vi "SysDef.Create.vi"(8 "error in (no error)":errorcluster, 10 "Configuration":T1={"Name"="", "Description"="", "Diagnostics Basic Configuraiton"={"CAN Interface"=enum."CAN0", "Baud Rate"=0, "Diagnostic Protocol"=enum."GMLAN", "Transport Protocol"=enum."ISO TP - Normal Mode", "Transmit ID"=0, "Receive ID"=0, "Transmit Extension"=0, "Receive Extension"=0, "Receive UUDT ID"=0, "Enable Stream"=TRUE, "VW TP Channel ID"=0, "Security"={"Source DLL Path"=path "", "Security Level"=1, "Target DLL Path"=path ""}, "Fill Frame"=FALSE, "Fill Byte"=255, "Termination"=FALSE}, "DID Outputs"={"Description"="", "Frames"=[]}, "DID Inputs"={"Description"="", "Frames"=[]}, "PID Outputs"={"Description"="", "Frames"=[]}, "PID Inputs"={"Description"="", "Frames"=[]}, "DPIDs"={"Description"="", "DPIDs"=[]}, "DTC"={"Description"="", "DTC descriptor"={"DTC Byte Length"=2, "Status Byte Length"=1, "Add Data Byte Length"=1, "Byte Order"=enum."Motorola"}, "DTC Control"={"Description"="", "Signals"=[]}, "Created DTCs"=0}, "NI 986x Support"={"Enable"=FALSE, "RIO Device"=0, "Bitfile"=path ""}, "Commands"={"Description"=""}, "Status"={"Description"=""}, "IO Controls"={"Description"="", "IO Control Array"=[]}, "Routines"={"Description"="", "Routine Array"=[]}, "Memory Outputs"={"Description"="", "Frames"=[]}, "Memory Inputs"={"Description"="", "Frames"=[]}, "User Defined"={"Description"="", "Groups"=[]}} {"DID Outputs"."Frames"."Signals"."Byte Order" items=["Little Endian", "Big Endian"]; "DID Outputs"."Frames"."Signals"."Data Type" items=["Signed", "Unsigned", "IEEE Float"]; "Memory Inputs"."Frames"."Signals"."Byte Order" items=["Little Endian", "Big Endian"]; "Memory Inputs"."Frames"."Signals"."Data Type" items=["Signed", "Unsigned", "IEEE Float"]; "Memory Outputs"."Frames"."Signals"."Byte Order" items=["Little Endian", "Big Endian"]; "Memory Outputs"."Frames"."Signals"."Data Type" items=["Signed", "Unsigned", "IEEE Float"]; "Routines"."Routine Array"."Stop Parameters"."Response"."Byte Order" items=["Little Endian", "Big Endian"]; "Routines"."Routine Array"."Stop Parameters"."Response"."Data Type" items=["Signed", "Unsigned", "IEEE Float"]; "Routines"."Routine Array"."Stop Parameters"."Cmd"."Byte Order" items=["Little Endian", "Big Endian"]; "Routines"."Routine Array"."Stop Parameters"."Cmd"."Data Type" items=["Signed", "Unsigned", "IEEE Float"]; "Routines"."Routine Array"."Request Parameters"."Response"."Byte Order" items=["Little Endian", "Big Endian"]; "Routines"."Routine Array"."Request Parameters"."Response"."Data Type" items=["Signed", "Unsigned", "IEEE Float"]; "Routines"."Routine Array"."Request Parameters"."Cmd"."Byte Order" items=["Little Endian", "Big Endian"]; "Routines"."Routine Array"."Request Parameters"."Cmd"."Data Type" items=["Signed", "Unsigned", "IEEE Float"]; "Routines"."Routine Array"."Start Parameters"."Response"."Byte Order" items=["Little Endian", "Big Endian"]; "Routines"."Routine Array"."Start Parameters"."Response"."Data Type" items=["Signed", "Unsigned", "IEEE Float"]; "Routines"."Routine Array"."Start Parameters"."Cmd"."Byte Order" items=["Little Endian", "Big Endian"]; "Routines"."Routine Array"."Start Parameters"."Cmd"."Data Type" items=["Signed", "Unsigned", "IEEE Float"]; "IO Controls"."IO Control Array"."Signals"."Response"."Byte Order" items=["Little Endian", "Big Endian"]; "IO Controls"."IO Control Array"."Signals"."Response"."Data Type" items=["Signed", "Unsigned", "IEEE Float"]; "IO Controls"."IO Control Array"."Signals"."Cmd"."Byte Order" items=["Little Endian", "Big Endian"]; "IO Controls"."IO Control Array"."Signals"."Cmd"."Data Type" items=["Signed", "Unsigned", "IEEE Float"]; "DTC"."DTC Control"."Signals"."Byte Order" items=["Little Endian", "Big Endian"]; "DTC"."DTC Control"."Signals"."Data Type" items=["Signed", "Unsigned", "IEEE Float"]; "Diagnostics Basic Configuraiton"."Fill Byte" format="%.0x"; "Diagnostics Basic Configuraiton"."VW TP Channel ID" format="%.0x"; "Diagnostics Basic Configuraiton"."Receive UUDT ID" format="%.0x"; "Diagnostics Basic Configuraiton"."Receive Extension" format="%.0x"; "Diagnostics Basic Configuraiton"."Transmit Extension" format="%.0x"; "Diagnostics Basic Configuraiton"."Receive ID" format="%.0x"; "Diagnostics Basic Configuraiton"."Transmit ID" format="%.0x"; "DID Inputs"."Frames"."Signals"."Byte Order" items=["Little Endian", "Big Endian"]; "DID Inputs"."Frames"."Signals"."Data Type" items=["Signed", "Unsigned", "IEEE Float"]; "PID Inputs"."Frames"."Signals"."Byte Order" items=["Little Endian", "Big Endian"]; "PID Inputs"."Frames"."Signals"."Data Type" items=["Signed", "Unsigned", "IEEE Float"]; "PID Outputs"."Frames"."Signals"."Byte Order" items=["Little Endian", "Big Endian"]; "PID Outputs"."Frames"."Signals"."Data Type" items=["Signed", "Unsigned", "IEEE Float"]}, 11 "Device Item Ref in":T28 format="%.0x") -> (0 "error out":errorcluster, 3 "Device Item Ref out":T28 format="%.0x")   [LabVIEW 2015, in "Diagnostics Addon System Explorer.lvlib"]
uses:
  Diagnostics Addon System Explorer.lvlib
  <vilib>/NI Veristand/Custom Device API/Custom Device Item Ref.ctl
  Types/SysDef.Export.ctl
  Shared/Types/CAN.ctl
  Shared/Types/CAN.Interface.ctl
  Shared/Types/Protocol.ctl
  Shared/Types/Transport.ctl
  Shared/Types/Security.ctl
  Types/Frames.Export.ctl
  Types/Frame.Export.ctl
  Shared/Types/Signal.ctl
  Types/DPIDs.Export.ctl
  Types/DPID.Export.ctl
  Shared/Types/DPID.ctl
  Shared/Types/DPID.Rate.ctl
  Types/DTC.Export.ctl
  Shared/Types/DTCDescriptor.ctl
  Types/DTCControl.Export.ctl
  Shared/Types/986x.ctl
  Types/Command.Export.ctl
  Types/Status.Export.ctl
  Types/IOControls.Export.ctl
  Types/IO.Export.ctl
  Types/CmdResp.Export.ctl
  Types/Routines.Export.ctl
  Types/Routine.Export.ctl
  Types/UserDefined.Export.ctl
  Types/UserDefined.Group.Export.ctl
  Types/UserDefined.Group.Message.Export.ctl
  Types/FG.Action.ctl
  <vilib>/NI Veristand/Custom Device API/Custom Device Channel.ctl
  <vilib>/NI Veristand/Custom Device API/Custom Device Channel Type.ctl
  Shared/Types/Type.ctl
  FileDependency.Create.vi
  Name.Create.vi
  ID.FG.vi
  ReadSignal.Create.vi
  <vilib>/NI Veristand/Custom Device API/NI VeriStand - Get Item Property.vi
  <vilib>/NI Veristand/Custom Device API/Get Item Property (U32).vi
  <vilib>/NI Veristand/Custom Device API/NI VeriStand - Set Item Property.vi
  <vilib>/NI Veristand/Custom Device API/Set Item Property (U32).vi
  Shared/SubVIs/Constants.vi
  <vilib>/NI Veristand/Custom Device API/Get Item Property (I32).vi
  <vilib>/NI Veristand/Custom Device API/Set Item Property (I32).vi
  <vilib>/NI Veristand/Custom Device API/Set Item Property (Boolean).vi
  <vilib>/NI Veristand/Custom Device API/NI VeriStand - Remove Item Property.vi
  <vilib>/NI Veristand/Custom Device API/Set Item Property (Dependent File).vi
  <vilib>/Utility/MD5Checksum.llb/MD5Checksum File.vi
  <vilib>/NI Veristand/Custom Device API/Get Item Property (Boolean).vi
  FileDependency.Get.Target Path.vi
  <vilib>/NI Veristand/Custom Device API/Custom Device API.lvlib
  Shared/Diagnostics Addon Shared.lvlib
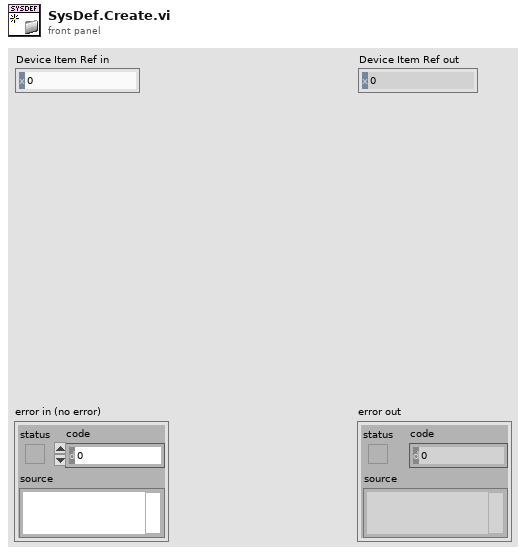
[diagram p1: front panel]
types:
  T1 = typedef "Diagnostics Addon System Explorer.lvlib/SysDef.Export.ctl" = cluster{"Name":string, "Description":string, "Diagnostics Basic Configuraiton":T2, "DID Outputs":T7, "DID Inputs":T7, "PID Outputs":T7, "PID Inputs":T7, "DPIDs":T10, "DTC":T14, "NI 986x Support":T17, "Commands":T18, "Status":T19, "IO Controls":T20, "Routines":T23, "Memory Outputs":T7, "Memory Inputs":T7, "User Defined":T25}
  T2 = typedef "Diagnostics Addon Shared.lvlib/CAN.ctl" = cluster{"CAN Interface":T3, "Baud Rate":u32, "Diagnostic Protocol":T4, "Transport Protocol":T5, "Transmit ID":u32, "Receive ID":u32, "Transmit Extension":u8, "Receive Extension":u8, "Receive UUDT ID":u32, "Enable Stream":bool, "VW TP Channel ID":u32, "Security":T6, "Fill Frame":bool, "Fill Byte":u8, "Termination":bool}
  T3 = typedef "Diagnostics Addon Shared.lvlib/CAN.Interface.ctl" = enum16{"CAN0", "CAN1", "CAN2", "CAN3", "CAN4", "CAN5", "CAN6", "CAN7", "CAN8", "CAN9", "CAN10", "CAN11", "CAN12", "CAN13", "CAN14", "CAN15", "CAN16", "CAN17", "CAN18", "CAN19", "CAN20", "CAN21", "CAN22", "CAN23", "CAN24", "CAN25", "CAN26", "CAN27", "CAN28", "CAN29", "CAN30", "CAN31", "CAN32", "CAN33", "CAN34", "CAN35", "CAN36", "CAN37", "CAN38", "CAN39", "CAN40", "CAN41", "CAN42", "CAN43", "CAN44", "CAN45", "CAN46", "CAN47", "CAN48", "CAN49", "CAN50", "CAN51", "CAN52", "CAN53", "CAN54", "CAN55", "CAN56", "CAN57", "CAN58", "CAN59", "CAN60", "CAN61", "CAN62", "CAN63", "CAN 256 (Virtual)", "CAN 257 (Virtual)"}
  T4 = typedef "Diagnostics Addon Shared.lvlib/Protocol.ctl" = enum16{"GMLAN", "KWP-2000", "UDS", "User-Defined"}
  T5 = typedef "Diagnostics Addon Shared.lvlib/Transport.ctl" = enum16{"ISO TP - Normal Mode", "ISO TP - Mixed Mode", "VW TP 2.0", "Diagnostics on IP"}
  T6 = typedef "Diagnostics Addon Shared.lvlib/Security.ctl" = cluster{"Source DLL Path":path, "Security Level":u8, "Target DLL Path":path}
  T7 = typedef "Diagnostics Addon System Explorer.lvlib/Frames.Export.ctl" = cluster{"Description":string, "Frames":T8[]}
  T8 = typedef "Diagnostics Addon System Explorer.lvlib/Frame.Export.ctl" = cluster{"Name":string, "Description":string, "ID":u32, "Signals":T9[]}
  T9 = typedef "Diagnostics Addon Shared.lvlib/Signal.ctl" = cluster{"Start Bit":u32, "Length":u32, "Scaling Factor":dbl, "Scaling Offset":dbl, "Minimum":dbl, "Maximum":dbl, "Data Type":u32, "Byte Order":u32, "Default Value":dbl, "Name":string, "Units":string, "Description":string}
  T10 = typedef "Diagnostics Addon System Explorer.lvlib/DPIDs.Export.ctl" = cluster{"Description":string, "DPIDs":T11[]}
  T11 = typedef "Diagnostics Addon System Explorer.lvlib/DPID.Export.ctl" = cluster{"Name":string, "Description":string, "DPID":T12}
  T12 = typedef "Diagnostics Addon Shared.lvlib/DPID.ctl" = cluster{"DPID ID":u8, "Speed":T13, "PIDs":u16[]}
  T13 = typedef "Diagnostics Addon Shared.lvlib/DPID.Rate.ctl" = enum16{"Slow", "Medium", "Fast"}
  T14 = typedef "Diagnostics Addon System Explorer.lvlib/DTC.Export.ctl" = cluster{"Description":string, "DTC descriptor":T15, "DTC Control":T16, "Created DTCs":u32}
  T15 = typedef "Diagnostics Addon Shared.lvlib/DTCDescriptor.ctl" = cluster{"DTC Byte Length":i32, "Status Byte Length":i32, "Add Data Byte Length":i32, "Byte Order":enum16{"Motorola", "Intel"}}
  T16 = typedef "Diagnostics Addon System Explorer.lvlib/DTCControl.Export.ctl" = cluster{"Description":string, "Signals":T9[]}
  T17 = typedef "Diagnostics Addon Shared.lvlib/986x.ctl" = cluster{"Enable":bool, "RIO Device":u16, "Bitfile":path}
  T18 = typedef "Diagnostics Addon System Explorer.lvlib/Command.Export.ctl" = cluster{"Description":string}
  T19 = typedef "Diagnostics Addon System Explorer.lvlib/Status.Export.ctl" = cluster{"Description":string}
  T20 = typedef "Diagnostics Addon System Explorer.lvlib/IOControls.Export.ctl" = cluster{"Description":string, "IO Control Array":T21[]}
  T21 = typedef "Diagnostics Addon System Explorer.lvlib/IO.Export.ctl" = cluster{"Name":string, "Description":string, "ID":u16, "Signals":T22}
  T22 = typedef "Diagnostics Addon System Explorer.lvlib/CmdResp.Export.ctl" = cluster{"Cmd":T9[], "Response":T9[]}
  T23 = typedef "Diagnostics Addon System Explorer.lvlib/Routines.Export.ctl" = cluster{"Description":string, "Routine Array":T24[]}
  T24 = typedef "Diagnostics Addon System Explorer.lvlib/Routine.Export.ctl" = cluster{"Name":string, "Description":string, "ID":u16, "Start Parameters":T22, "Request Parameters":T22, "Stop Parameters":T22}
  T25 = typedef "Diagnostics Addon System Explorer.lvlib/UserDefined.Export.ctl" = cluster{"Description":string, "Groups":T26[]}
  T26 = typedef "Diagnostics Addon System Explorer.lvlib/UserDefined.Group.Export.ctl" = cluster{"Name":string, "Description":string, "Messages":T27[]}
  T27 = typedef "Diagnostics Addon System Explorer.lvlib/UserDefined.Group.Message.Export.ctl" = cluster{"Name":string, "Description":string, "Signals":T22}
  T28 = typedef "Custom Device API.lvlib/Custom Device Item Ref.ctl" = u64
  T29 = typedef "Diagnostics Addon System Explorer.lvlib/FG.Action.ctl" = enum16{"Get", "Set"}
  T30 = typedef "Custom Device API.lvlib/Custom Device Channel.ctl" = cluster{"Type":T31, "Units":string, "Default Value":dbl, "Faultable":bool, "Scalable":bool}
  T31 = typedef "Custom Device API.lvlib/Custom Device Channel Type.ctl" = enum16{"Input", "Output"}
  T32 = typedef "Diagnostics Addon Shared.lvlib/Type.ctl" = enum16{"DID", "CDID", "PID", "CPID", "Read Memory", "Write Memory", "DTC Control", "IO Cmd", "IO Resp", "Routine Start Cmd", "Routine Start Resp", "Routine Request Cmd", "Routine Request Resp", "Routine Stop Cmd", "Routine Stop Resp", "UserDefined Cmd", "UserDefined Rsp"}
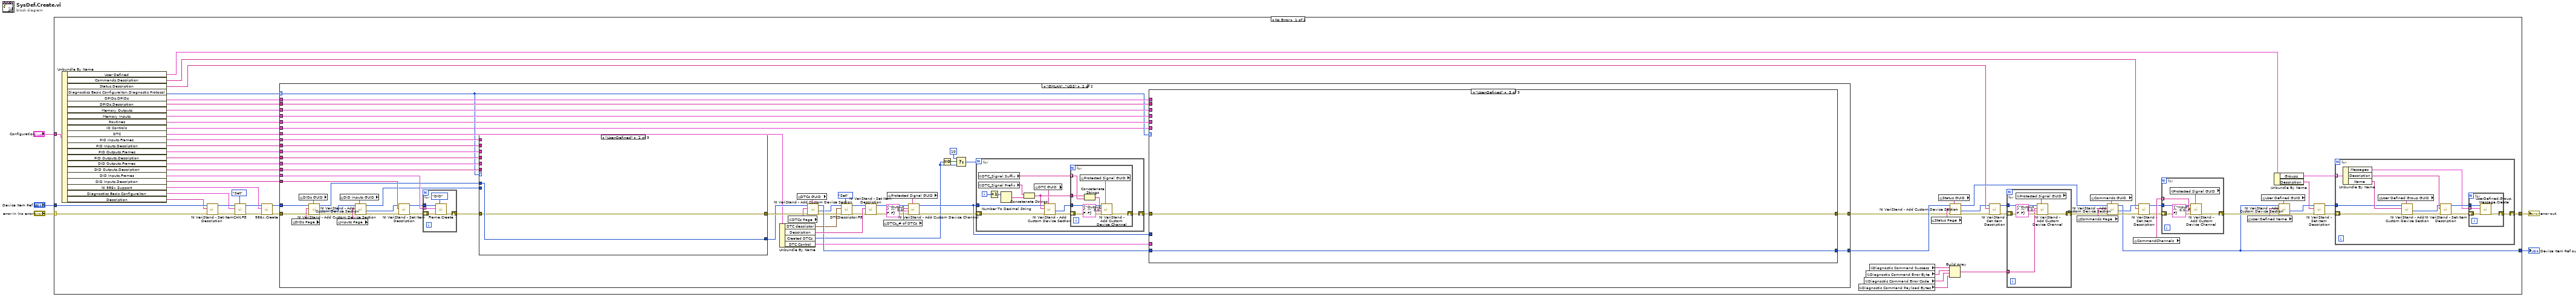
[diagram p0: block diagram]
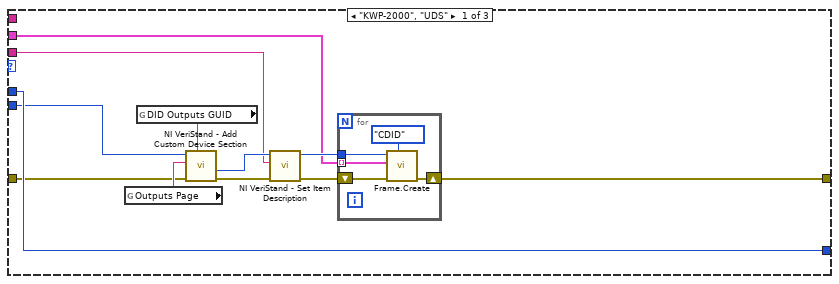
[diagram p3: hidden frame]
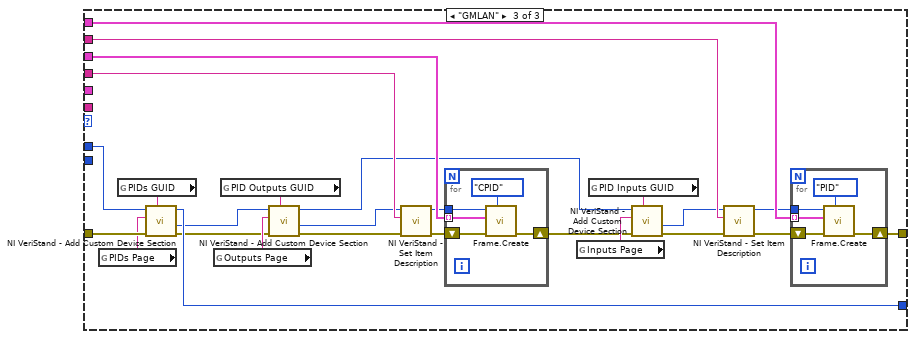
[diagram p4: hidden frame]
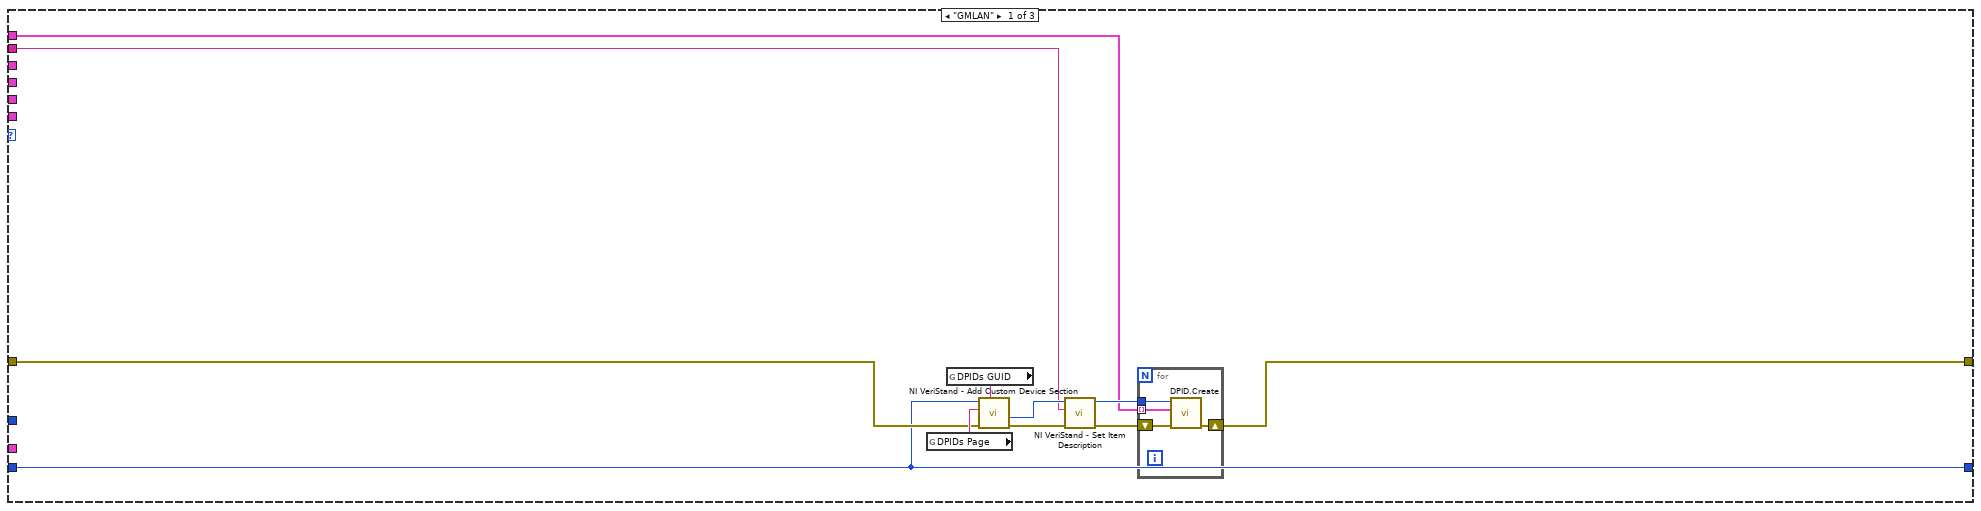
[diagram p5: hidden frame]
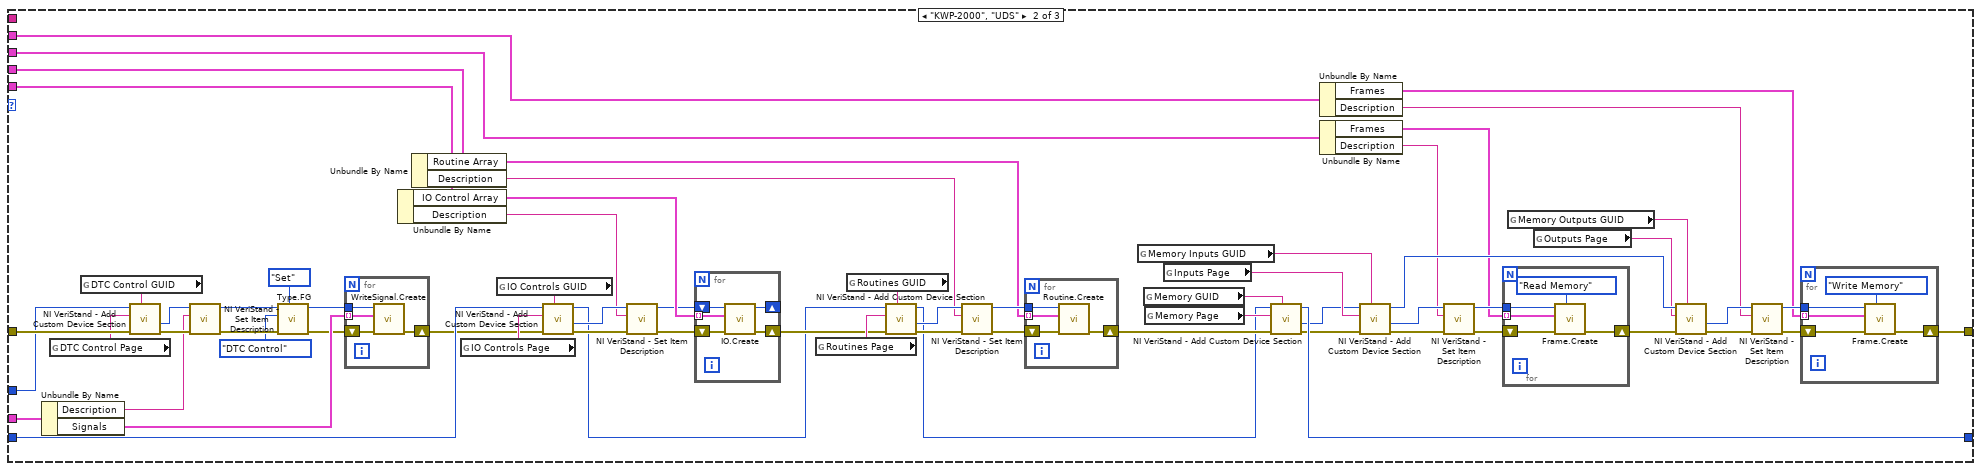
[diagram p6: hidden frame]
diagram:
  n1 = case shown="No Error" "error in (no error)" {
    selector: "error in (no error)" -> [w60 w345]
    tunnel: [w9 w345] -> w4
    tunnel: "Device Item Ref in" -> [w64 w344]
    tunnel: [w12 w344] -> w2
    tunnel: "Configuration" -> [w63 _]
    frame No Error {
      n2 = Unbundle By Name(w63) -> ("User Defined"=w18:T25, "Commands.Description"=w44:string, "Status.Description"=w45:string, "Diagnostics Basic Configuraiton.Diagnostic Protocol"=w6:T4, "DPIDs.DPIDs"=w22:T11[], "DPIDs.Description"=w21:string, "Memory Outputs"=w35:T7, "Memory Inputs"=w34:T7, "Routines"=w36:T23, "IO Controls"=w37:T20, "DTC"=w50:T14, "PID Inputs.Frames"=w52:T8[], "PID Inputs.Description"=w53:string, "PID Outputs.Frames"=w51:T8[], "PID Outputs.Description"=w54:string, "DID Outputs.Frames"=w20:T8[], "DID Outputs.Description"=w19:string, "DID Inputs.Frames"=w55:T8[], "DID Inputs.Description"=w56:string, "NI 986x Support"=w39:T17, "Diagnostics Basic Configuraiton"=w58:T2, "Description"=w59:string)
      n3 = call <vilib>:"NI VeriStand - Set Item Description.vi"("error in (no error)"=w60, "Description"=w59, "Item Ref in"=w64) -> ("error out"=w61:errorcluster, "Item Ref out"=w62:T28)  [unwired: 6 in, 1 out]
      n4 = call "CAN.FG.vi"("Action"=FG.Action."Set", "error in (no error)"=w61, "Diagnostics Basic Configuraiton"=w58, "Device Item Ref in"=w62) -> ("error out"=w43:errorcluster, "Device Item Ref out"=w40:T28)  [unwired: 5 in, 1 out]
      n5 = call "986x.Create.vi"("error in (no error)"=w43, "986x Support"=w39, "Device Item Ref in"=w40) -> ("error out"=w42:errorcluster, "Device Ref out"=w41:T28)  [unwired: 7 in]
      n6 = case shown="\"GMLAN\"..\"UDS\"" w6 {
        selector: w6 -> [_ w78]
        tunnel: w56 -> [_ w120]
        tunnel: w55 -> [_ w119]
        tunnel: w54 -> [_ w118]
        tunnel: w53 -> [_ w117]
        tunnel: w52 -> [_ w116]
        tunnel: w51 -> [_ w115]
        tunnel: w50 -> [_ w114]
        tunnel: w42 -> [w72 w110]
        tunnel: w41 -> [w71 w109]
        tunnel: [w71 w106] -> w38
        tunnel: w37 -> [_ w77]
        tunnel: w36 -> [_ w105]
        tunnel: w35 -> [_ w104]
        tunnel: w34 -> [_ w103]
        tunnel: [w72 w83] -> w23
        tunnel: w22 -> [_ w82]
        tunnel: w21 -> [_ w81]
        tunnel: w20 -> [_ w80]
        tunnel: w19 -> [_ w79]
        frame "User-Defined" {
        }
        frame "GMLAN".."UDS" {
          n7 = global read "Constants.vi" "DIDs Page"() -> (w94:string)
          n8 = global read "Constants.vi" "DIDs GUID"() -> (w93:string)
          n9 = call <vilib>:"NI VeriStand - Add Custom Device Section.vi"("GUID (Default Section)"=w93, "error in (no error)"=w110, "Section Name"=w94, "Parent Ref in"=w109) -> ("error out"=w86:errorcluster, "Section Ptr"=w85:T28, "Parent Ref out"=w122:T28)  [unwired: 4 in, 1 out]
          n10 = global read "Constants.vi" "Inputs Page"() -> (w91:string)
          n11 = global read "Constants.vi" "DID Inputs GUID"() -> (w92:string)
          n12 = call <vilib>:"NI VeriStand - Add Custom Device Section.vi"("GUID (Default Section)"=w92, "error in (no error)"=w86, "Section Name"=w91, "Parent Ref in"=w85) -> ("error out"=w90:errorcluster, "Section Ptr"=w89:T28, "Parent Ref out"=w84:T28)  [unwired: 4 in, 1 out]
          n13 = call <vilib>:"NI VeriStand - Set Item Description.vi"("error in (no error)"=w90, "Description"=w120, "Item Ref in"=w89) -> ("error out"=w88:errorcluster, "Item Ref out"=w87:T28)  [unwired: 6 in, 1 out]
          n14 = for {
            tunnel: w87 -> [w188]
            shift-right: [w187] -> w123
            shift-left: w88 -> [w190]
            tunnel: w119 -> [w189] mode=indexing
            n15 = call "Frame.Create.vi"("Type"=Type."DID", "error in (no error)"=w190, "Frame"=w189, "Section Ptr"=w188) -> ("error out"=w187:errorcluster)  [unwired: 6 in, 1 out]
          }
          n16 = case shown="\"User-Defined\"" w78 {
            tunnel: [w137 w148 w175] -> w128
            tunnel: [w136 w149 w174] -> w127
            tunnel: w123 -> [w135 w148 w173]
            tunnel: w122 -> [w136 w149 w172]
            tunnel: w118 -> [_ _ w171]
            tunnel: w117 -> [_ _ w170]
            tunnel: w116 -> [_ _ w169]
            tunnel: w115 -> [_ _ w168]
            tunnel: w84 -> [w134 _ _]
            tunnel: w80 -> [w131 _ _]
            tunnel: w79 -> [w132 _ _]
            frame "KWP-2000", "UDS" {
              n17 = global read "Constants.vi" "Outputs Page"() -> (w142:string)
              n18 = global read "Constants.vi" "DID Outputs GUID"() -> (w133:string)
              n19 = call <vilib>:"NI VeriStand - Add Custom Device Section.vi"("GUID (Default Section)"=w133, "error in (no error)"=w135, "Section Name"=w142, "Parent Ref in"=w134) -> ("error out"=w141:errorcluster, "Section Ptr"=w140:T28)  [unwired: 4 in, 2 out]
              n20 = call <vilib>:"NI VeriStand - Set Item Description.vi"("error in (no error)"=w141, "Description"=w132, "Item Ref in"=w140) -> ("error out"=w138:errorcluster, "Item Ref out"=w139:T28)  [unwired: 6 in, 1 out]
              n21 = for {
                tunnel: w139 -> [w145]
                shift-right: [w146] -> w137
                shift-left: w138 -> [w147]
                tunnel: w131 -> [w144] mode=indexing
                n22 = call "Frame.Create.vi"("Type"=Type."CDID", "error in (no error)"=w147, "Frame"=w144, "Section Ptr"=w145) -> ("error out"=w146:errorcluster)  [unwired: 6 in, 1 out]
              }
            }
            frame "User-Defined" {
            }
            frame "GMLAN" {
              n23 = global read "Constants.vi" "PIDs Page"() -> (w166:string)
              n24 = global read "Constants.vi" "PIDs GUID"() -> (w167:string)
              n25 = call <vilib>:"NI VeriStand - Add Custom Device Section.vi"("GUID (Default Section)"=w167, "error in (no error)"=w173, "Section Name"=w166, "Parent Ref in"=w172) -> ("error out"=w161:errorcluster, "Section Ptr"=w160:T28, "Parent Ref out"=w174:T28)  [unwired: 4 in, 1 out]
              n26 = global read "Constants.vi" "Outputs Page"() -> (w162:string)
              n27 = global read "Constants.vi" "PID Outputs GUID"() -> (w163:string)
              n28 = call <vilib>:"NI VeriStand - Add Custom Device Section.vi"("GUID (Default Section)"=w163, "error in (no error)"=w161, "Section Name"=w162, "Parent Ref in"=w160) -> ("error out"=w159:errorcluster, "Section Ptr"=w154:T28, "Parent Ref out"=w150:T28)  [unwired: 4 in, 1 out]
              n29 = call <vilib>:"NI VeriStand - Set Item Description.vi"("error in (no error)"=w159, "Description"=w171, "Item Ref in"=w154) -> ("error out"=w152:errorcluster, "Item Ref out"=w153:T28)  [unwired: 6 in, 1 out]
              n30 = for {
                tunnel: w153 -> [w178]
                shift-right: [w179] -> w151
                shift-left: w152 -> [w180]
                tunnel: w168 -> [w177] mode=indexing
                n31 = call "Frame.Create.vi"("Type"=Type."CPID", "error in (no error)"=w180, "Frame"=w177, "Section Ptr"=w178) -> ("error out"=w179:errorcluster)  [unwired: 6 in, 1 out]
              }
              n32 = global read "Constants.vi" "Inputs Page"() -> (w164:string)
              n33 = global read "Constants.vi" "PID Inputs GUID"() -> (w165:string)
              n34 = call <vilib>:"NI VeriStand - Add Custom Device Section.vi"("GUID (Default Section)"=w165, "error in (no error)"=w151, "Section Name"=w164, "Parent Ref in"=w150) -> ("error out"=w158:errorcluster, "Section Ptr"=w156:T28)  [unwired: 4 in, 2 out]
              n35 = call <vilib>:"NI VeriStand - Set Item Description.vi"("error in (no error)"=w158, "Description"=w170, "Item Ref in"=w156) -> ("error out"=w157:errorcluster, "Item Ref out"=w155:T28)  [unwired: 6 in, 1 out]
              n36 = for {
                tunnel: w155 -> [w183]
                shift-right: [w184] -> w175
                shift-left: w157 -> [w185]
                tunnel: w169 -> [w182] mode=indexing
                n37 = call "Frame.Create.vi"("Type"=Type."PID", "error in (no error)"=w185, "Frame"=w182, "Section Ptr"=w183) -> ("error out"=w184:errorcluster)  [unwired: 6 in, 1 out]
              }
            }
          }
          n38 = Unbundle By Name(w114) -> ("DTC descriptor"=w97:T15, "Description"=w111:string, "Created DTCs"=w75:u32, "DTC Control"=w95:T16)
          n39 = global read "Constants.vi" "DTCs Page"() -> (w130:string)
          n40 = global read "Constants.vi" "DTCs GUID"() -> (w129:string)
          n41 = call <vilib>:"NI VeriStand - Add Custom Device Section.vi"("GUID (Default Section)"=w129, "error in (no error)"=w128, "Section Name"=w130, "Parent Ref in"=w127) -> ("error out"=w101:errorcluster, "Section Ptr"=w102:T28, "Parent Ref out"=w107:T28)  [unwired: 4 in, 1 out]
          n42 = call "DTCDescriptor.FG.vi"("Action"=FG.Action."Set", "error in (no error)"=w101, "DTC descriptor"=w97, "Device Item Ref in"=w102) -> ("error out"=w100:errorcluster, "Device Item Ref out"=w99:T28)  [unwired: 5 in, 1 out]
          n43 = call <vilib>:"NI VeriStand - Set Item Description.vi"("error in (no error)"=w100, "Description"=w111, "Item Ref in"=w99) -> ("error out"=w113:errorcluster, "Item Ref out"=w112:T28)  [unwired: 6 in, 1 out]
          n44 = global read "Constants.vi" "DTCs_# of DTCs"() -> (w125:string)
          n45 = global read "Constants.vi" "Protected Signal GUID"() -> (w121:string)
          n46 = call <vilib>:"NI VeriStand - Add Custom Device Channel.vi"("GUID (Default Channel)"=w121, "error in (no error)"=w113, "Channel"=T30 {"Type"=enum."Output", "Units"="", "Default Value"=0.0, "Faultable"=FALSE, "Scalable"=FALSE}, "Channel Name"=w125, "Parent Ref in"=w112) -> ("error out"=w124:errorcluster, "Parent Ref out"=w96:T28)  [unwired: 3 in, 2 out]
          n47 = Equal To 0?(x=w75) -> (x = 0?=w76:bool)
          n48 = Select(t=u32 10, s=w76, f=w75) -> (s? t:f=w74:u32)
          n49 = for {
            N: w74 -> [_]
            tunnel: w96 -> [w303]
            shift-right: [w307] -> w108
            shift-left: w124 -> [w301]
            i -> [w306]
            n50 = global read "Constants.vi" "DTC_Signal Suffix"() -> (w298:string[])
            n51 = global read "Constants.vi" "DTC_Signal Prefix"() -> (w297:string)
            n52 = Increment(x=w306) -> (x+1=w305:i32)
            n53 = Number To Decimal String(number=w305) -> (decimal integer string=w304:string)  [unwired: 1 in]
            n54 = Concatenate Strings(w297, w304) -> (w299:string)
            n55 = global read "Constants.vi" "DTC GUID"() -> (w296:string)
            n56 = call <vilib>:"NI VeriStand - Add Custom Device Section.vi"("GUID (Default Section)"=w296, "error in (no error)"=w301, "Section Name"=w299, "Parent Ref in"=w303) -> ("error out"=w300:errorcluster, "Section Ptr"=w302:T28)  [unwired: 4 in, 2 out]
            n57 = for {
              tunnel: w302 -> [w313]
              tunnel: w299 -> [w310]
              tunnel: w298 -> [w311] mode=indexing
              shift-right: [w315] -> w307
              shift-left: w300 -> [w312]
              n58 = global read "Constants.vi" "Protected Signal GUID"() -> (w308:string)
              n59 = Concatenate Strings(w310, w311) -> (w309:string)
              n60 = call <vilib>:"NI VeriStand - Add Custom Device Channel.vi"("GUID (Default Channel)"=w308, "error in (no error)"=w312, "Channel"=T30 {"Type"=enum."Output", "Units"="", "Default Value"=0.0, "Faultable"=FALSE, "Scalable"=FALSE}, "Channel Name"=w309, "Parent Ref in"=w313) -> ("error out"=w315:errorcluster)  [unwired: 3 in, 3 out]
            }
          }
          n61 = case shown="\"User-Defined\"" w78 {
            tunnel: w108 -> [w195 w221 w295]
            tunnel: w107 -> [w193 w257 w294]
            tunnel: [w193 w245 w294] -> w106
            tunnel: [w194 w230 w295] -> w83
            tunnel: w77 -> [_ w265 _]
            tunnel: w105 -> [_ w252 _]
            tunnel: w104 -> [_ w224 _]
            tunnel: w103 -> [_ w227 _]
            tunnel: w96 -> [_ w220 _]
            tunnel: w95 -> [_ w215 _]
            tunnel: w82 -> [w191 _ _]
            tunnel: w81 -> [w192 _ _]
            frame "GMLAN" {
              n62 = global read "Constants.vi" "DPIDs Page"() -> (w200:string)
              n63 = global read "Constants.vi" "DPIDs GUID"() -> (w201:string)
              n64 = call <vilib>:"NI VeriStand - Add Custom Device Section.vi"("GUID (Default Section)"=w201, "error in (no error)"=w195, "Section Name"=w200, "Parent Ref in"=w193) -> ("error out"=w199:errorcluster, "Section Ptr"=w197:T28)  [unwired: 4 in, 2 out]
              n65 = call <vilib>:"NI VeriStand - Set Item Description.vi"("error in (no error)"=w199, "Description"=w192, "Item Ref in"=w197) -> ("error out"=w198:errorcluster, "Item Ref out"=w196:T28)  [unwired: 6 in, 1 out]
              n66 = for {
                tunnel: w196 -> [w203]
                shift-right: [w204] -> w194
                shift-left: w198 -> [w205]
                tunnel: w191 -> [w202] mode=indexing
                n67 = call "DPID.Create.vi"("error in (no error)"=w205, "DPID"=w202, "Section Ptr"=w203) -> ("error out"=w204:errorcluster)  [unwired: 7 in, 1 out]
              }
            }
            frame "KWP-2000", "UDS" {
              n68 = Unbundle By Name(w215) -> ("Description"=w214:string, "Signals"=w213:T9[])
              n69 = global read "Constants.vi" "DTC Control Page"() -> (w212:string)
              n70 = global read "Constants.vi" "DTC Control GUID"() -> (w211:string)
              n71 = call <vilib>:"NI VeriStand - Add Custom Device Section.vi"("GUID (Default Section)"=w211, "error in (no error)"=w221, "Section Name"=w212, "Parent Ref in"=w220) -> ("error out"=w216:errorcluster, "Section Ptr"=w218:T28)  [unwired: 4 in, 2 out]
              n72 = call <vilib>:"NI VeriStand - Set Item Description.vi"("error in (no error)"=w216, "Description"=w214, "Item Ref in"=w218) -> ("error out"=w209:errorcluster, "Item Ref out"=w217:T28)  [unwired: 6 in, 1 out]
              n73 = call "Type.FG.vi"("Action"=FG.Action."Set", "error in (no error)"=w209, "Type"=Type."DTC Control", "Device Item Ref in"=w217) -> ("error out"=w208:errorcluster, "Device Item Ref out"=w210:T28)  [unwired: 5 in, 1 out]
              n74 = for {
                shift-right: [w273] -> w219
                shift-left: w208 -> [w274]
                tunnel: w213 -> [w272] mode=indexing
                tunnel: w210 -> [w271]
                n75 = call "WriteSignal.Create.vi"("error in (no error)"=w274, "Signal Parameters"=w272, "Section Ptr"=w271) -> ("error out"=w273:errorcluster)  [unwired: 7 in, 1 out]
              }
              n76 = Unbundle By Name(w265) -> ("IO Control Array"=w264:T21[], "Description"=w255:string)
              n77 = Unbundle By Name(w252) -> ("Routine Array"=w251:T24[], "Description"=w250:string)
              n78 = global read "Constants.vi" "IO Controls Page"() -> (w262:string)
              n79 = global read "Constants.vi" "IO Controls GUID"() -> (w263:string)
              n80 = call <vilib>:"NI VeriStand - Add Custom Device Section.vi"("GUID (Default Section)"=w263, "error in (no error)"=w219, "Section Name"=w262, "Parent Ref in"=w257) -> ("error out"=w261:errorcluster, "Section Ptr"=w260:T28, "Parent Ref out"=w256:T28)  [unwired: 4 in, 1 out]
              n81 = call <vilib>:"NI VeriStand - Set Item Description.vi"("error in (no error)"=w261, "Description"=w255, "Item Ref in"=w260) -> ("error out"=w259:errorcluster, "Item Ref out"=w258:T28)  [unwired: 6 in, 1 out]
              n82 = for {
                shift-right: [w292] -> w266
                shift-left: w259 -> [w293]
                shift-right: [w290] -> _
                shift-left: w258 -> [w291]
                tunnel: w264 -> [w289] mode=indexing
                n83 = call "IO.Create.vi"("error in (no error)"=w293, "IO Control"=w289, "Section Ptr"=w291) -> ("error out"=w292:errorcluster, "Parent Ref out"=w290:T28)  [unwired: 7 in]
              }
              n84 = global read "Constants.vi" "Routines Page"() -> (w268:string)
              n85 = global read "Constants.vi" "Routines GUID"() -> (w267:string)
              n86 = call <vilib>:"NI VeriStand - Add Custom Device Section.vi"("GUID (Default Section)"=w267, "error in (no error)"=w266, "Section Name"=w268, "Parent Ref in"=w256) -> ("error out"=w269:errorcluster, "Section Ptr"=w270:T28, "Parent Ref out"=w246:T28)  [unwired: 4 in, 1 out]
              n87 = call <vilib>:"NI VeriStand - Set Item Description.vi"("error in (no error)"=w269, "Description"=w250, "Item Ref in"=w270) -> ("error out"=w254:errorcluster, "Item Ref out"=w253:T28)  [unwired: 6 in, 1 out]
              n88 = for {
                shift-right: [w287] -> w247
                shift-left: w254 -> [w288]
                tunnel: w253 -> [w286]
                tunnel: w251 -> [w285] mode=indexing
                n89 = call "Routine.Create.vi"("error in (no error)"=w288, "Routine"=w285, "Section Ptr"=w286) -> ("error out"=w287:errorcluster)  [unwired: 7 in, 1 out]
              }
              n90 = global read "Constants.vi" "Memory Inputs GUID"() -> (w244:string)
              n91 = global read "Constants.vi" "Memory GUID"() -> (w249:string)
              n92 = global read "Constants.vi" "Memory Page"() -> (w248:string)
              n93 = global read "Constants.vi" "Inputs Page"() -> (w243:string)
              n94 = call <vilib>:"NI VeriStand - Add Custom Device Section.vi"("GUID (Default Section)"=w249, "error in (no error)"=w247, "Section Name"=w248, "Parent Ref in"=w246) -> ("error out"=w229:errorcluster, "Section Ptr"=w228:T28, "Parent Ref out"=w245:T28)  [unwired: 4 in, 1 out]
              n95 = Unbundle By Name(w224) -> ("Frames"=w223:T8[], "Description"=w222:string)
              n96 = Unbundle By Name(w227) -> ("Frames"=w225:T8[], "Description"=w226:string)
              n97 = call <vilib>:"NI VeriStand - Add Custom Device Section.vi"("GUID (Default Section)"=w244, "error in (no error)"=w229, "Section Name"=w243, "Parent Ref in"=w228) -> ("error out"=w242:errorcluster, "Section Ptr"=w237:T28, "Parent Ref out"=w233:T28)  [unwired: 4 in, 1 out]
              n98 = call <vilib>:"NI VeriStand - Set Item Description.vi"("error in (no error)"=w242, "Description"=w226, "Item Ref in"=w237) -> ("error out"=w235:errorcluster, "Item Ref out"=w236:T28)  [unwired: 6 in, 1 out]
              n99 = for {
                tunnel: w236 -> [w277]
                shift-right: [w278] -> w234
                shift-left: w235 -> [w279]
                tunnel: w225 -> [w276] mode=indexing
                n100 = call "Frame.Create.vi"("Type"=Type."Read Memory", "error in (no error)"=w279, "Frame"=w276, "Section Ptr"=w277) -> ("error out"=w278:errorcluster)  [unwired: 6 in, 1 out]
              }
              n101 = global read "Constants.vi" "Memory Outputs GUID"() -> (w231:string)
              n102 = global read "Constants.vi" "Outputs Page"() -> (w232:string)
              n103 = call <vilib>:"NI VeriStand - Add Custom Device Section.vi"("GUID (Default Section)"=w231, "error in (no error)"=w234, "Section Name"=w232, "Parent Ref in"=w233) -> ("error out"=w241:errorcluster, "Section Ptr"=w239:T28)  [unwired: 4 in, 2 out]
              n104 = call <vilib>:"NI VeriStand - Set Item Description.vi"("error in (no error)"=w241, "Description"=w222, "Item Ref in"=w239) -> ("error out"=w240:errorcluster, "Item Ref out"=w238:T28)  [unwired: 6 in, 1 out]
              n105 = for {
                tunnel: w238 -> [w282]
                shift-right: [w283] -> w230
                shift-left: w240 -> [w284]
                tunnel: w223 -> [w281] mode=indexing
                n106 = call "Frame.Create.vi"("Type"=Type."Write Memory", "error in (no error)"=w284, "Frame"=w281, "Section Ptr"=w282) -> ("error out"=w283:errorcluster)  [unwired: 6 in, 1 out]
              }
            }
            frame "User-Defined" {
            }
          }
        }
      }
      n107 = global read "Constants.vi" "Diagnostic Command Payload Bytes"() -> (w25:string)
      n108 = global read "Constants.vi" "Diagnostic Command Error Code"() -> (w24:string)
      n109 = global read "Constants.vi" "Diagnostic Command Error Byte"() -> (w27:string)
      n110 = global read "Constants.vi" "Diagnostic Command Success"() -> (w28:string)
      n111 = global read "Constants.vi" "Status Page"() -> (w69:string)
      n112 = global read "Constants.vi" "Status GUID"() -> (w70:string)
      n113 = Build Array(w28, w27, w24, w25) -> (w26:string[])
      n114 = call <vilib>:"NI VeriStand - Add Custom Device Section.vi"("GUID (Default Section)"=w70, "error in (no error)"=w23, "Section Name"=w69, "Parent Ref in"=w38) -> ("error out"=w30:errorcluster, "Section Ptr"=w29:T28, "Parent Ref out"=w66:T28)  [unwired: 4 in, 1 out]
      n115 = call <vilib>:"NI VeriStand - Set Item Description.vi"("error in (no error)"=w30, "Description"=w45, "Item Ref in"=w29) -> ("error out"=w33:errorcluster, "Item Ref out"=w32:T28)  [unwired: 6 in, 1 out]
      n116 = for {
        tunnel: w32 -> [w335]
        shift-right: [w334] -> w31
        shift-left: w33 -> [w336]
        tunnel: w26 -> [w333] mode=indexing
        n117 = global read "Constants.vi" "Protected Signal GUID"() -> (w332:string)
        n118 = call <vilib>:"NI VeriStand - Add Custom Device Channel.vi"("GUID (Default Channel)"=w332, "error in (no error)"=w336, "Channel"=T30 {"Type"=enum."Output", "Units"="", "Default Value"=0.0, "Faultable"=FALSE, "Scalable"=FALSE}, "Channel Name"=w333, "Parent Ref in"=w335) -> ("error out"=w334:errorcluster)  [unwired: 3 in, 3 out]
      }
      n119 = global read "Constants.vi" "Commands Page"() -> (w68:string)
      n120 = global read "Constants.vi" "Commands GUID"() -> (w67:string)
      n121 = call <vilib>:"NI VeriStand - Add Custom Device Section.vi"("GUID (Default Section)"=w67, "error in (no error)"=w31, "Section Name"=w68, "Parent Ref in"=w66) -> ("error out"=w49:errorcluster, "Section Ptr"=w47:T28, "Parent Ref out"=w12:T28)  [unwired: 4 in, 1 out]
      n122 = global read "Constants.vi" "CommandChannels"() -> (w65:string[])
      n123 = call <vilib>:"NI VeriStand - Set Item Description.vi"("error in (no error)"=w49, "Description"=w44, "Item Ref in"=w47) -> ("error out"=w48:errorcluster, "Item Ref out"=w46:T28)  [unwired: 6 in, 1 out]
      n124 = for {
        tunnel: w65 -> [w343] mode=indexing
        tunnel: w46 -> [w341]
        shift-right: [w339] -> w13
        shift-left: w48 -> [w342]
        n125 = global read "Constants.vi" "Protected Signal GUID"() -> (w338:string)
        n126 = call <vilib>:"NI VeriStand - Add Custom Device Channel.vi"("GUID (Default Channel)"=w338, "error in (no error)"=w342, "Channel"=T30 {"Type"=enum."Input", "Units"="", "Default Value"=0.0, "Faultable"=FALSE, "Scalable"=FALSE}, "Channel Name"=w343, "Parent Ref in"=w341) -> ("error out"=w339:errorcluster)  [unwired: 3 in, 3 out]
      }
      n127 = global read "Constants.vi" "User Defined Name"() -> (w14:string)
      n128 = global read "Constants.vi" "User Defined GUID"() -> (w15:string)
      n129 = Unbundle By Name(w18) -> ("Groups"=w7:T26[], "Description"=w11:string)
      n130 = call <vilib>:"NI VeriStand - Add Custom Device Section.vi"("GUID (Default Section)"=w15, "error in (no error)"=w13, "Section Name"=w14, "Parent Ref in"=w12) -> ("error out"=w16:errorcluster, "Section Ptr"=w17:T28)  [unwired: 4 in, 2 out]
      n131 = call <vilib>:"NI VeriStand - Set Item Description.vi"("error in (no error)"=w16, "Description"=w11, "Item Ref in"=w17) -> ("error out"=w10:errorcluster, "Item Ref out"=w8:T28)  [unwired: 6 in, 1 out]
      n132 = for {
        tunnel: w8 -> [w323]
        shift-right: [w317] -> w9
        shift-left: w10 -> [w324]
        tunnel: w7 -> [w326] mode=indexing
        n133 = Unbundle By Name(w326) -> ("Messages"=w316:T27[], "Description"=w320:string, "Name"=w325:string)
        n134 = global read "Constants.vi" "User Defined Group GUID"() -> (w327:string)
        n135 = call <vilib>:"NI VeriStand - Add Custom Device Section.vi"("GUID (Default Section)"=w327, "error in (no error)"=w324, "Section Name"=w325, "Parent Ref in"=w323) -> ("error out"=w321:errorcluster, "Section Ptr"=w322:T28)  [unwired: 4 in, 2 out]
        n136 = call <vilib>:"NI VeriStand - Set Item Description.vi"("error in (no error)"=w321, "Description"=w320, "Item Ref in"=w322) -> ("error out"=w318:errorcluster, "Item Ref out"=w319:T28)  [unwired: 6 in, 1 out]
        n137 = for {
          tunnel: w319 -> [w331]
          tunnel: w316 -> [w328] mode=indexing
          shift-right: [w329] -> w317
          shift-left: w318 -> [w330]
          n138 = call "UserDefined.Group.Message.Create.vi"("error in (no error)"=w330, "Message"=w328, "Section Ptr"=w331) -> ("error out"=w329:errorcluster)  [unwired: 7 in, 1 out]
        }
      }
    }
    frame Error {
    }
  }
  "error out" <- w4
  "Device Item Ref out" <- w2
